vi "truncate.vi"(11 "Array in":dbl[](array[numeric])) -> (3 "Array out":dbl[](array[numeric]))   [LabVIEW 2016]
doc: "truncates beginning of array if over 10000 elements"
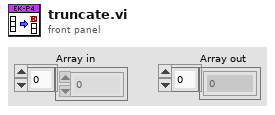
[diagram p1: front panel]
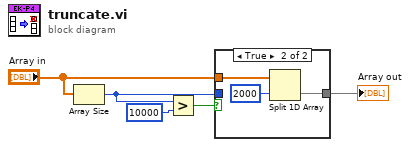
[diagram p0: block diagram]
diagram:
  n1 = Array Size(array="Array in") -> (size(s)=w4:i32)
  n2 = Greater?(x=w4, y=10000) -> (0:w2:bool)
  n3 = case shown="True" w2 {
    tunnel: "Array in" -> [w6 w9]
    tunnel: w4 -> [_ _]
    tunnel: [w6 w8] -> w5
    frame False {
    }
    frame True {
      n4 = Split 1D Array(array=w9, index=2000) -> (second subarray=w8:dbl[])  [unwired: 1 out]
    }
  }
  "Array out" <- w5
